vi "Make Canonical Query String.vi"(11 "request parameters":cluster{"item":string, "value":string}[](array[cluster])) -> (3 "canonical parameters":string)   [LabVIEW 2015, in "NI_AWS Core.lvlib"]
uses:
  NI_AWS Core.lvlib
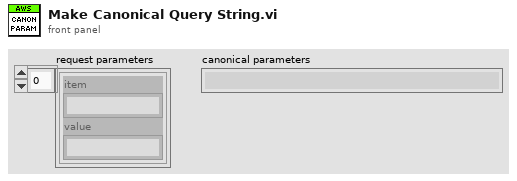
[diagram p1: front panel]
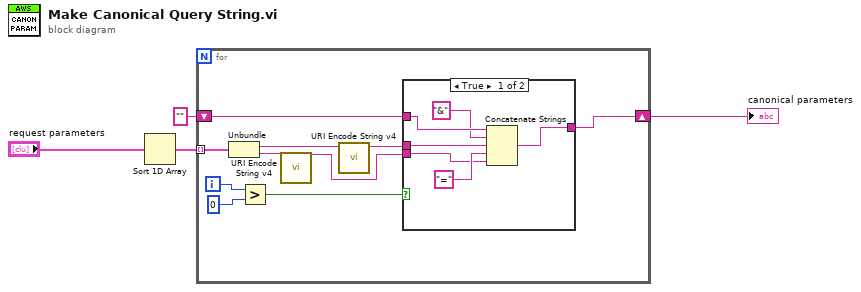
[diagram p0: block diagram]
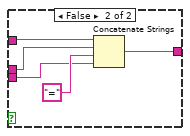
[diagram p2: hidden frame]
diagram:
  n1 = Sort 1D Array(array="request parameters") -> (sorted array=w3:cluster{"item":string, "value":string}[])
  n2 = for {
    tunnel: w3 -> [w14] mode=indexing
    shift-right: [w11] -> w1
    shift-left: "" -> [w12]
    i -> [w9]
    n3 = Unbundle(w14) -> ("item"=w7:string, "value"=w8:string)
    n4 = Greater?(x=w9, y=0 ("x")) -> (0:w13:bool)
    n5 = call "URI Encode String v4.vi"("Un-encoded String"=w8) -> ("UriEncoded String"=w5:string)  [unwired: 10 in]
    n6 = call "URI Encode String v4.vi"("Un-encoded String"=w7) -> ("UriEncoded String"=w6:string)  [unwired: 10 in]
    n7 = case shown="True" w13 {
      tunnel: w12 -> [w20 w21]
      tunnel: w6 -> [w18 w25]
      tunnel: w5 -> [w16 w23]
      tunnel: [w15 w22] -> w11
      frame True {
        n8 = Concatenate Strings(w20, "&" ("string"), w18, "=" ("string"), w16) -> (w15:string)
      }
      frame False {
        n9 = Concatenate Strings(w21, w25, "=" ("string"), w23) -> (w22:string)
      }
    }
  }
  "canonical parameters" <- w1
